vi "TSLIN_SendRespond.vi"(8 "错误输入":errorcluster, 9 "Data":T2 {"REC_Channel" items=["CHN1", "CHN2", "CHN3", "CHN4", "CHN5", "CHN6", "CHN7", "CHN8", "CHN9", "CHN10", "CHN11", "CHN12", "CHN13", "CHN14", "CHN15", "CHN16", "CHN17", "CHN18", "CHN19", "CHN20", "CHN21", "CHN22", "CHN23", "CHN24", "CHN25", "CHN26", "CHN27", "CHN28", "CHN29", "CHN30", "CHN31", "CHN32"]; "LIN_Data"."REC_Channel" items=["CHN1", "CHN2", "CHN3", "CHN4", "CHN5", "CHN6", "CHN7", "CHN8", "CHN9", "CHN10", "CHN11", "CHN12", "CHN13", "CHN14", "CHN15", "CHN16", "CHN17", "CHN18", "CHN19", "CHN20", "CHN21", "CHN22", "CHN23", "CHN24", "CHN25", "CHN26", "CHN27", "CHN28", "CHN29", "CHN30", "CHN31", "CHN32"]; "LIN_Data"."LIN Scheduling Table Array"."LIN_Transmit"."Channel" items=["CHN1", "CHN2", "CHN3", "CHN4", "CHN5", "CHN6", "CHN7", "CHN8", "CHN9", "CHN10", "CHN11", "CHN12", "CHN13", "CHN14", "CHN15", "CHN16", "CHN17", "CHN18", "CHN19", "CHN20", "CHN21", "CHN22", "CHN23", "CHN24", "CHN25", "CHN26", "CHN27", "CHN28", "CHN29", "CHN30", "CHN31", "CHN32"]; "LIN_Data"."LIN Scheduling Table Array"."LIN_Transmit"."ID" format="%.0x"; "LIN_Data"."LIN Scheduling Table Array"."LIN_Transmit"."DLC" format="%.0x"; "LIN_Data"."LIN Scheduling Table Array"."LIN_Transmit"."Set_node_funtiontype" items=["MasterNode", "SlaveNode", "MonitorNote"]; "LIN_Data"."LDF"."LDF loading channel" items=["CHN1", "CHN2", "CHN3", "CHN4", "CHN5", "CHN6", "CHN7", "CHN8", "CHN9", "CHN10", "CHN11", "CHN12", "CHN13", "CHN14", "CHN15", "CHN16", "CHN17", "CHN18", "CHN19", "CHN20", "CHN21", "CHN22", "CHN23", "CHN24", "CHN25", "CHN26", "CHN27", "CHN28", "CHN29", "CHN30", "CHN31", "CHN32"]; "LIN_Data"."LIN_Set_Array"."Set_node_funtiontype" items=["MasterNode", "SlaveNode", "MonitorNote"]; "LIN_Data"."LIN_Set_Array"."Set"."Hardware Type" items=["BUS_UNKNOWN_TYPE", "TS_TCP_DEVICE", "XL_USB_DEVICE", "TS_USB_DEVICE", "PEAK_USB_DEVICE", "KVASER_USB_DEVICE", "ZLG_USB_DEVICE", "ICS_USB_DEVICE", "TS_TC1005_DEVICE", "CANABLE_USB_DEVICE", "TS_WIRELESS_OBD", "TS_USB_DEVICE_EX", "IXXAT_USB_DEVICE", "TS_ETH_IF_DEVICE", "TS_USB_IF_DEVICE", "BUS_DEV_TYPE_COUNT"]; "LIN_Data"."LIN_Set_Array"."Set"."AHwChannel" items=["CHN1", "CHN2", "CHN3", "CHN4", "CHN5", "CHN6", "CHN7", "CHN8", "CHN9", "CHN10", "CHN11", "CHN12", "CHN13", "CHN14", "CHN15", "CHN16", "CHN17", "CHN18", "CHN19", "CHN20", "CHN21", "CHN22", "CHN23", "CHN24", "CHN25", "CHN26", "CHN27", "CHN28", "CHN29", "CHN30", "CHN31", "CHN32"]; "LIN_Data"."LIN_Set_Array"."Set"."AAppChannel" items=["CHN1", "CHN2", "CHN3", "CHN4", "CHN5", "CHN6", "CHN7", "CHN8", "CHN9", "CHN10", "CHN11", "CHN12", "CHN13", "CHN14", "CHN15", "CHN16", "CHN17", "CHN18", "CHN19", "CHN20", "CHN21", "CHN22", "CHN23", "CHN24", "CHN25", "CHN26", "CHN27", "CHN28", "CHN29", "CHN30", "CHN31", "CHN32"]; "LIN_Data"."LIN_Set_Array"."Set"."AProtocol" items=["Lin_Protocol_13", "Lin_Protocol_20", "Lin_Protocol_21", "Lin_Protocol_J2602"]; "LIN_Data"."Funtiontype" items=["MasterNode", "SlaveNode", "MonitorNote"]; "LIN_Data"."LIN_SendHead"."ALINDLC" format="%.0x"; "LIN_Data"."LIN_SendHead"."ALINId" format="%.0x"; "LIN_Data"."LIN_SendHead"."ALINIdxchn" items=["CHN1", "CHN2", "CHN3", "CHN4", "CHN5", "CHN6", "CHN7", "CHN8", "CHN9", "CHN10", "CHN11", "CHN12", "CHN13", "CHN14", "CHN15", "CHN16", "CHN17", "CHN18", "CHN19", "CHN20", "CHN21", "CHN22", "CHN23", "CHN24", "CHN25", "CHN26", "CHN27", "CHN28", "CHN29", "CHN30", "CHN31", "CHN32"]; "LIN_Data"."LIN_Set"."Hardware Type" items=["BUS_UNKNOWN_TYPE", "TS_TCP_DEVICE", "XL_USB_DEVICE", "TS_USB_DEVICE", "PEAK_USB_DEVICE", "KVASER_USB_DEVICE", "ZLG_USB_DEVICE", "ICS_USB_DEVICE", "TS_TC1005_DEVICE", "CANABLE_USB_DEVICE", "TS_WIRELESS_OBD", "TS_USB_DEVICE_EX", "IXXAT_USB_DEVICE", "TS_ETH_IF_DEVICE", "TS_USB_IF_DEVICE", "BUS_DEV_TYPE_COUNT"]; "LIN_Data"."LIN_Set"."AHwChannel" items=["CHN1", "CHN2", "CHN3", "CHN4", "CHN5", "CHN6", "CHN7", "CHN8", "CHN9", "CHN10", "CHN11", "CHN12", "CHN13", "CHN14", "CHN15", "CHN16", "CHN17", "CHN18", "CHN19", "CHN20", "CHN21", "CHN22", "CHN23", "CHN24", "CHN25", "CHN26", "CHN27", "CHN28", "CHN29", "CHN30", "CHN31", "CHN32"]; "LIN_Data"."LIN_Set"."AAppChannel" items=["CHN1", "CHN2", "CHN3", "CHN4", "CHN5", "CHN6", "CHN7", "CHN8", "CHN9", "CHN10", "CHN11", "CHN12", "CHN13", "CHN14", "CHN15", "CHN16", "CHN17", "CHN18", "CHN19", "CHN20", "CHN21", "CHN22", "CHN23", "CHN24", "CHN25", "CHN26", "CHN27", "CHN28", "CHN29", "CHN30", "CHN31", "CHN32"]; "LIN_Data"."LIN_Set"."AProtocol" items=["Lin_Protocol_13", "Lin_Protocol_20", "Lin_Protocol_21", "Lin_Protocol_J2602"]; "LIN_Data"."Channels used" items=["1 Channel"=1, "2 Channels"=2, "3 Channels"=3, "4 Channels"=4, "5 Channels"=5]}, 10 "ALINBuffer":T1[](array[typedef]), 11 "SendRespond":bool) -> (0 "error out":errorcluster, 2 "value":i32, 3 "succeed ?":bool)   [LabVIEW 2014]
uses:
  Typedef/TSLIN_Transmit.ctl
  Utilities/Typedef/Hardware_Subtype.ctl
  Typedef/TSLIN_SetData.ctl
  Typedef/TSLIN_SendHead.ctl
  Typedef/TSLIN_Config.ctl
  Typedef/TLibLIN.ctl
  Typedef/TSLIN_Data.ctl
  Typedef/TSLIN_LIN Schedule_Table.ctl
  Typedef/TSLIN_LIN_Set.ctl
  All_Control/Typedef/Hardware Type.ctl
  All_Control/Typedef/Blf_Log.ctl
  DataBase/Typedef/CAN/TCANSignal.ctl
  DataBase/Typedef/LIN/TLINSignal.ctl
  DataBase/Typedef/FlexRay/TFlexRaySignal.ctl
  DataBase/Typedef/TDBSignalProperties.ctl
  DataBase/Typedef/TDBFrameProperties.ctl
  DataBase/Typedef/TDBECUProperties.ctl
  DataBase/Typedef/TDBProperties.ctl
  DataBase/Typedef/DataBase_array.ctl
  DataBase/Typedef/DataBase_array_index.ctl
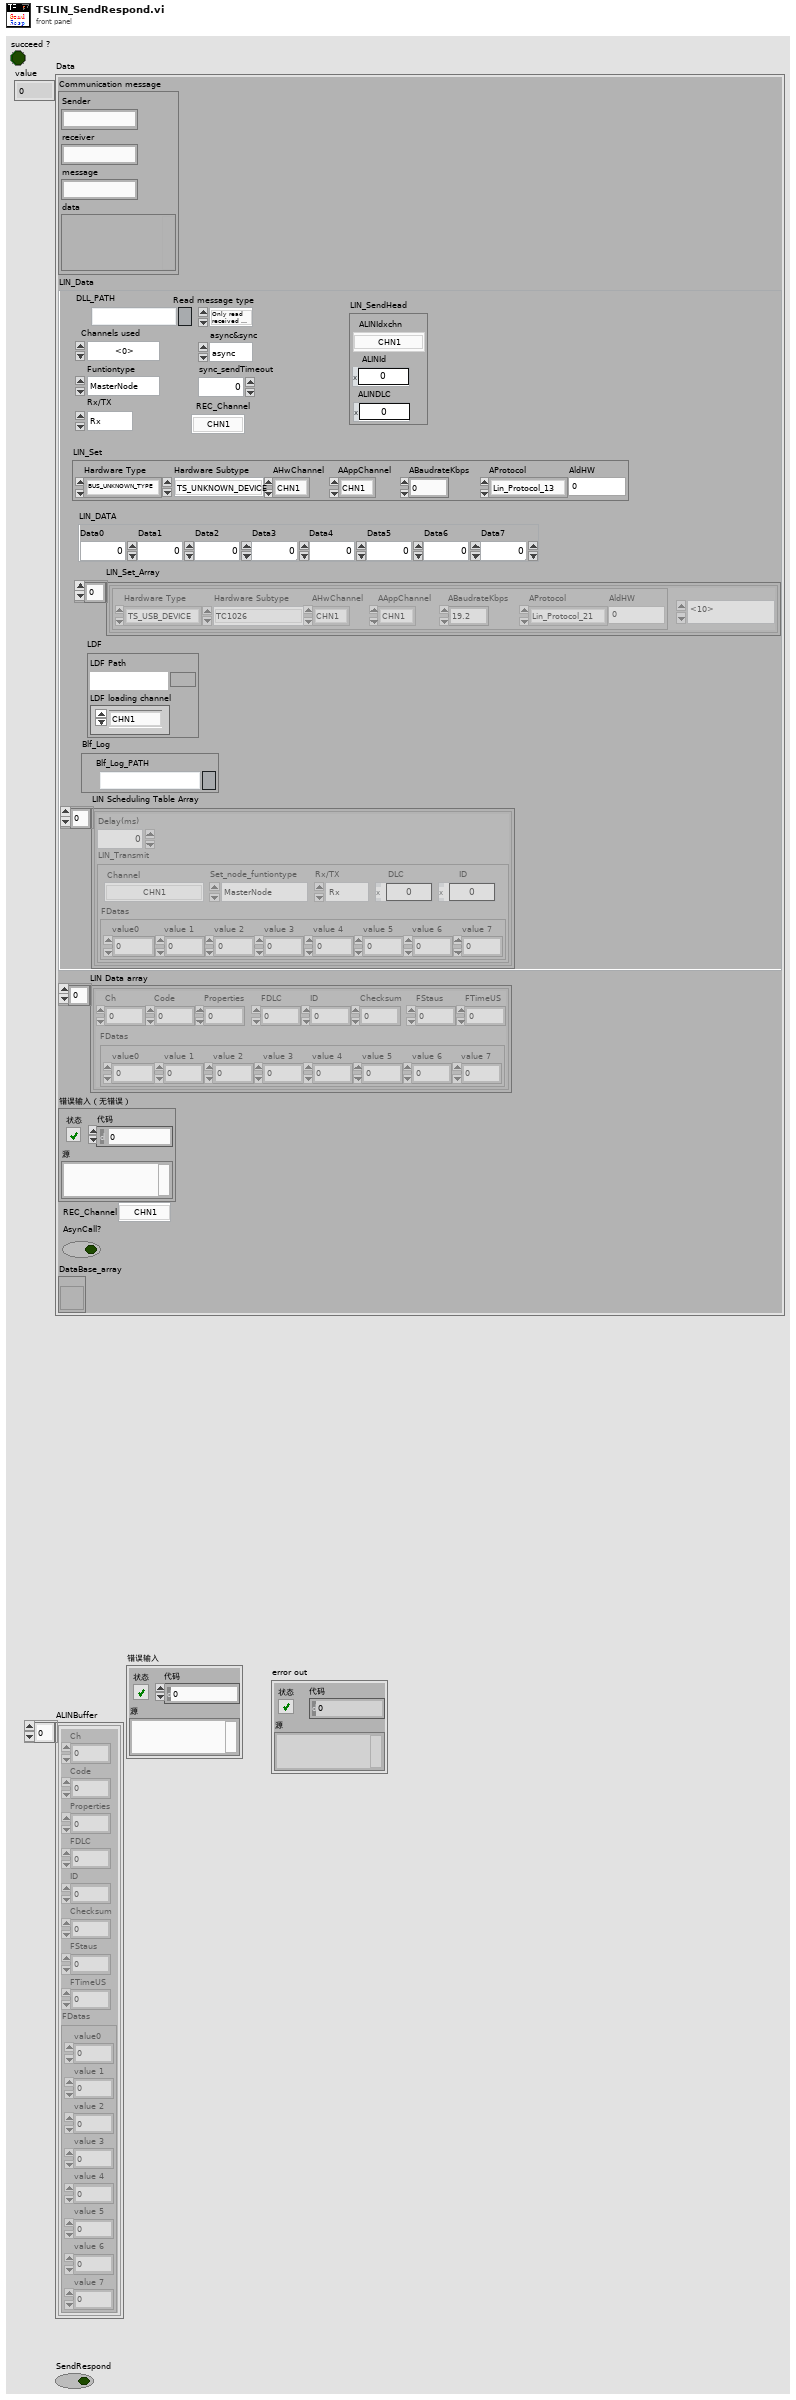
[diagram p1: front panel]
types:
  T1 = typedef "TLibLIN.ctl" = cluster{"Ch":u8, "Code":u8, "Properties":u8, "FDLC":u8, "ID":u8, "Checksum":u8, "FStaus":u8, "FTimeUS":u64, "FDatas":cluster{"value0":u8, "value 1":u8, "value 2":u8, "value 3":u8, "value 4":u8, "value 5":u8, "value 6":u8, "value 7":u8}}
  T2 = typedef "TSLIN_Data.ctl" = cluster{"Communication message":cluster{"Sender":string, "receiver":string, "message":string, "data":variant}, "LIN_Data":T3, "LIN Data array":T1[], "error in":errorcluster, "REC_Channel":i32, "AsynCall?":bool, "DataBase_array":T12}
  T3 = typedef "TSLIN_Config.ctl" = cluster{"DLL_PATH":path, "Channels used":u16, "Funtiontype":i32, "Rx/TX":enum16{"Rx", "Tx"}, "Read message type":enum16{"Only read received messages", "Receive&send messages"}, "async&sync":enum16{"async", "sync"}, "sync_sendTimeout":u16, "LIN_SendHead":T4, "LIN_Set":T5, "LIN_DATA":cluster{"Data0":u8, "Data1":u8, "Data2":u8, "Data3":u8, "Data4":u8, "Data5":u8, "Data6":u8, "Data7":u8}, "LIN_Set_Array":T8[], "LDF":cluster{"LDF Path":path, "LDF loading channel":i32}, "Blf_Log":T9, "LIN Scheduling Table Array":T10[], "REC_Channel":i32}
  T4 = typedef "TSLIN_SendHead.ctl" = cluster{"ALINIdxchn":u8, "ALINId":u32, "ALINDLC":u32}
  T5 = typedef "TSLIN_SetData.ctl" = cluster{"Hardware Type":T6, "Hardware Subtype":T7, "AHwChannel":i32, "AAppChannel":i32, "ABaudrateKbps":sgl, "AProtocol":i32, "AldHW":i32}
  T6 = typedef "Hardware Type.ctl" = i32
  T7 = typedef "Hardware_Subtype.ctl" = enum16{"TS_UNKNOWN_DEVICE", "TSCAN_PRO", "TSCAN_Lite1", "TC1001", "TL1001", "TC1011", "TM5011", "TC1002", "TC1014", "TSCANFD2517", "TC1026", "TC1016", "TC1012", "TC1013", "TLog1002", "TC1034", "TC1018", "GW2116", "TC2115", "MP1013", "TC1113", "TC1114", "TP1013", "TC1017", "TP1018", "TF10XX", "TL1004_FD_4_LIN_2", "TE1051", "TP1051", "TP1034", "TTS9015", "TP1026", "TTS1026", "TTS1034", "TTS1018", "TL1011", "TTS1015_LiAuto", "TTS1013_LiAuto", "TTS1016Pro", "TC1054Pro", "TC1054", "TLog1038", "TO1013", "TC1034Pro", "TC1018Pro", "TC1038Pro", "TS_DEV_END"}
  T8 = typedef "TSLIN_LIN_Set.ctl" = cluster{"Set":T5, "Set_node_funtiontype":i32}
  T9 = typedef "Blf_Log.ctl" = cluster{"Blf_Log_PATH":path}
  T10 = typedef "TSLIN_LIN Schedule_Table.ctl" = cluster{"LIN_Transmit":T11, "Delay(ms)":i32}
  T11 = typedef "TSLIN_Transmit.ctl" = cluster{"Channel":i32, "Rx/TX":enum16{"Rx", "Tx"}, "Set_node_funtiontype":i32, "DLC":u32, "ID":u32, "FDatas":cluster{"value0":u8, "value 1":u8, "value 2":u8, "value 3":u8, "value 4":u8, "value 5":u8, "value 6":u8, "value 7":u8}}
  T12 = typedef "DataBase_array_index.ctl" = refnum<vi>
  T13 = cluster{"Data0":u8, "Data1":u8, "Data2":u8, "Data3":u8, "Data4":u8, "Data5":u8, "Data6":u8, "Data7":u8}
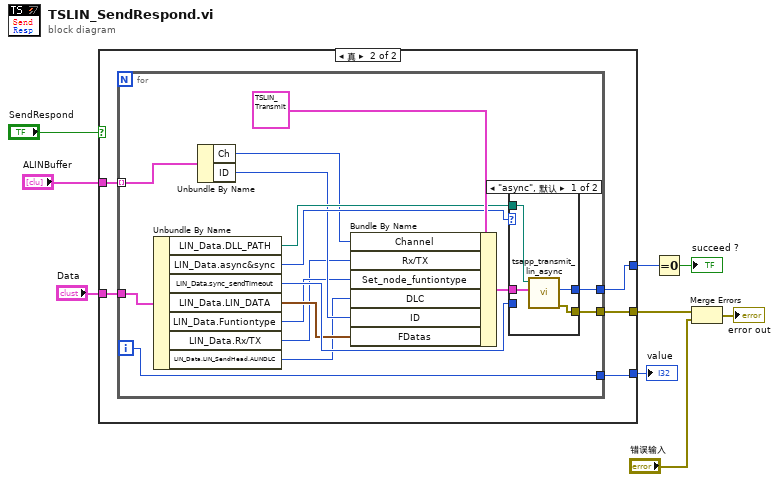
[diagram p0: block diagram]
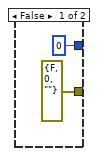
[diagram p2: hidden frame]
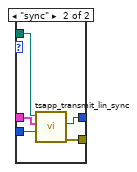
[diagram p3: hidden frame]
diagram:
  n1 = case shown="真" "SendRespond" {
    tunnel: "ALINBuffer" -> [_ w16]
    tunnel: "Data" -> [_ w15]
    tunnel: [errorcluster {"status"=FALSE, "code"=0, "source"=""} ("error out") w14] -> w5
    tunnel: [0 ("return") w13] -> w6
    tunnel: [_ w12] -> w2
    frame False {
    }
    frame True {
      n2 = for {
        tunnel: w16 -> [w32] mode=indexing
        tunnel: w15 -> [w29]
        tunnel: [w20] -> w13
        tunnel: [w19] -> w14
        tunnel: [w17] -> w12
        i -> [w17]
        n3 = Unbundle By Name(w29) -> ("LIN_Data.DLL_PATH"=w27:path, "LIN_Data.async&sync"=w28:enum16{"async", "sync"}, "LIN_Data.sync_sendTimeout"=w26:u16, "LIN_Data.LIN_DATA"=w24:T13, "LIN_Data.Funtiontype"=w22:i32, "LIN_Data.Rx/TX"=w21:enum16{"Rx", "Tx"}, "LIN_Data.LIN_SendHead.ALINDLC"=w18:u32)
        n4 = Unbundle By Name(w32) -> ("Ch"=w25:u8, "ID"=w23:u8)
        n5 = Bundle By Name(cluster=T11 {"Channel"=0, "Rx/TX"=enum."Rx", "Set_node_funtiontype"=0, "DLC"=0, "ID"=0, "FDatas"={"value0"=0, "value 1"=0, "value 2"=0, "value 3"=0, "value 4"=0, "value 5"=0, "value 6"=0, "value 7"=0}} ("LIN_Transmit"), "Channel"=w25, "Rx/TX"=w21, "Set_node_funtiontype"=w22, "DLC"=w18, "ID"=w23, "FDatas"=w24) -> (w30:T11)
        n6 = case shown="\"async\", 默认" w28 {
          tunnel: w30 -> [w36 w41]
          tunnel: w27 -> [w35 w40]
          tunnel: w26 -> [_ w39]
          tunnel: [w34 w38] -> w20
          tunnel: [w33 w37] -> w19
          frame "async", Default {
            n7 = call "tsapp_transmit_lin_async.vi"("LIN_Transmit"=w36, "Path"=w35) -> ("error out"=w33:errorcluster, "return"=w34:i32)  [unwired: 7 in, 1 out]
          }
          frame "sync" {
            n8 = call "tsapp_transmit_lin_sync.vi"("ATimeoutMS"=w39, "LIN_Transmit"=w41, "路径输入"=w40) -> ("错误输出"=w37:errorcluster, "return"=w38:i32)  [unwired: 6 in, 1 out]
          }
        }
      }
    }
  }
  "value" <- w2
  n9 = Equal To 0?(x=w6) -> (x = 0?=→"succeed ?":bool)
  n10 = Merge Errors(w5, "错误输入") -> (→"error out":errorcluster)
